vi "Straight Edge Detection subvi.vi"(8 "error in (no error)":errorcluster, 10 "ROI in":T2, 11 "Image in":T1(plugin-control)=refnum) -> (0 "error out":errorcluster, 1 "Solution Vector, y and x":dbl[](array[numeric]) format="%.2f", 2 "correct number of lines found = T":bool, 3 "Image":T1(plugin-control), 4 "edges found":i32)   [LabVIEW 2017]
doc: "This example shows how to use Find Straight Edges in NI Vision. Find Straight Edges finds lines (or straight edges) within a search region. Find Straight Edges is a precursor function to many of the gauging and inspection tasks. For example, the location of the straight edges found within a region that encloses an object can interpreted as the boundaries of the object whose dimensions have to be measured for a gauging application or the presence of a crack in the surface of an object for an inspection application."
uses:
  <vilib>/vision/NI_Vision_Development_Module.lvlib
panel:
  out "Straight Edges":T3(array[cluster])=[{"Point1 (Pixels)"={"X"=692.82367, "Y"=439.5}, "Point2 (Pixels)"={"X"=689.4538, "Y"=536.0}, "Point1 (Real-World)"={"X"=692.82367, "Y"=439.5}, "Point2 (Real-World)"={"X"=689.4538, "Y"=536.0}, "Angle (Pixel)"=-1.9999999999996223, "Angle (Real-World)"=-1.9999999999996223, "Score"=309.80392156862746, "Straightness"=0.0, "Average SNR (db)"=291.0237373163493, "Calibration Valid"=TRUE}, {"Point1 (Pixels)"={"X"=689.4637, "Y"=439.5}, "Point2 (Pixels)"={"X"=684.4063, "Y"=536.0}, "Point1 (Real-World)"={"X"=689.4637, "Y"=439.5}, "Point2 (Real-World)"={"X"=684.4063, "Y"=536.0}, "Angle (Pixel)"=-2.9999999999994333, "Angle (Real-World)"=-2.9999999999994333, "Score"=290.19607843137254, "Straightness"=0.0, "Average SNR (db)"=290.45582988516, "Calibration Valid"=TRUE}] {"Point2 (Real-World)"."Y" format="%.2f"; "Point2 (Real-World)"."X" format="%.2f"; "Point1 (Real-World)"."Y" format="%.2f"; "Point1 (Real-World)"."X" format="%.2f"; "Point2 (Pixels)"."Y" format="%.2f"; "Point2 (Pixels)"."X" format="%.2f"; "Point1 (Pixels)"."Y" format="%.2f"; "Point1 (Pixels)"."X" format="%.2f"}
  in  "Line Options":T4={"Number of Lines"=2, "Type"=4, "Minimum Score"=100.0, "Maximum Score"=1024.0, "Orientation"=0.0, "Angle Range"=10.0, "Angle Tolerance"=1.0, "Step Size"=3, "Min. SNR (db)"=0.0, "Min. Points (%)"=25.0, "Hough Iterations"=5} {"Min. Points (%)" min=0.0 max=100.0; "Min. SNR (db)" min=0.0; "Maximum Score" min=0.0 max=1024.0; "Minimum Score" min=1.0 max=1024.0 step=1.0; "Type" items=["First Edge Rake", "Best Edge Rake", "Hough Edge Rake", "First Edge Projection", "Best Edge Projection"]}
  in  "Edge Options":T5={"Edge Polarity"=0, "Kernel Size"=5, "Width"=3, "Minimum Edge Strength"=50.0, "Interpolation Type"=1, "Data Processing Method"=0} {"Data Processing Method" items=["Average", "Median"]; "Interpolation Type" items=["Zero Order"=0, "Bilinear"=1, "Bilinear Fixed"=4]; "Minimum Edge Strength" min=0.0 max=255.0 format="%.2g"; "Width" min=1 step=2; "Kernel Size" min=3 step=2; "Edge Polarity" items=["All Edges", "Rising Edges", "Falling Edges"]}
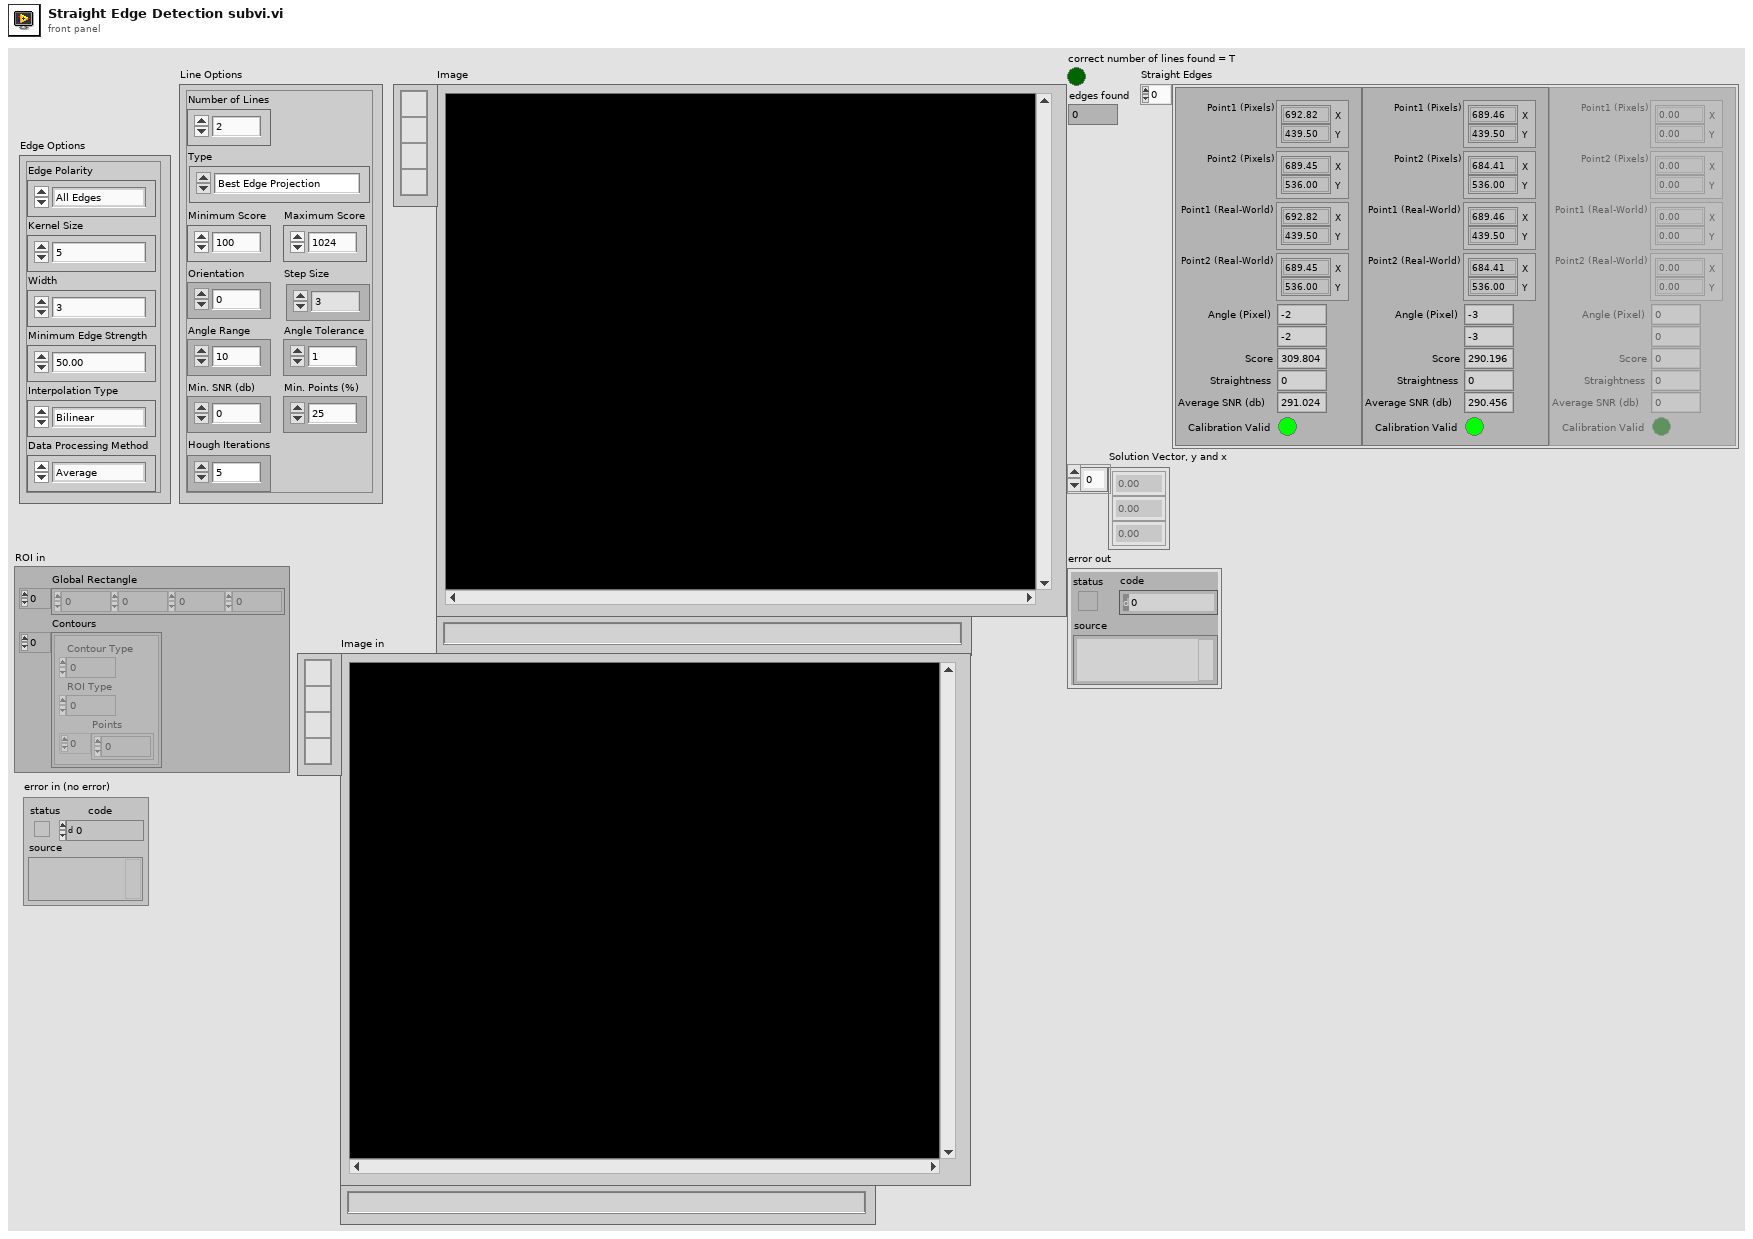
[diagram p1: front panel]
types:
  T1 = typedef "IMAQ Image.ctl" = refnum<image>
  T2 = cluster{"Global Rectangle":i32[], "Contours":cluster{"Contour Type":u32, "ROI Type":u32, "Points":i32[]}[]}
  T3 = cluster{"Point1 (Pixels)":cluster{"X":sgl, "Y":sgl}, "Point2 (Pixels)":cluster{"X":sgl, "Y":sgl}, "Point1 (Real-World)":cluster{"X":sgl, "Y":sgl}, "Point2 (Real-World)":cluster{"X":sgl, "Y":sgl}, "Angle (Pixel)":dbl, "Angle (Real-World)":dbl, "Score":dbl, "Straightness":dbl, "Average SNR (db)":dbl, "Calibration Valid":bool}[]
  T4 = cluster{"Number of Lines":i32, "Type":u16, "Minimum Score":dbl, "Maximum Score":dbl, "Orientation":dbl, "Angle Range":dbl, "Angle Tolerance":dbl, "Step Size":u32, "Min. SNR (db)":dbl, "Min. Points (%)":dbl, "Hough Iterations":i32}
  T5 = cluster{"Edge Polarity":u16, "Kernel Size":u32, "Width":u32, "Minimum Edge Strength":dbl, "Interpolation Type":u16, "Data Processing Method":u16}
  T6 = typedef "Search Line.ctl" = cluster{"Start Point":cluster{"X":sgl, "Y":sgl}, "End Point":cluster{"X":sgl, "Y":sgl}, "Edge Info":T7[], "Edge Map":dbl[], "Calibration Valid":bool}
  T7 = typedef "Edge New.ctl" = cluster{"Location (Pixel)":cluster{"X":sgl, "Y":sgl}, "Location (Real-World)":cluster{"X":sgl, "Y":sgl}, "Distance (Pixel)":dbl, "Distance (Real-World)":dbl, "Strength":dbl, "Noise":dbl, "Rising?":bool}
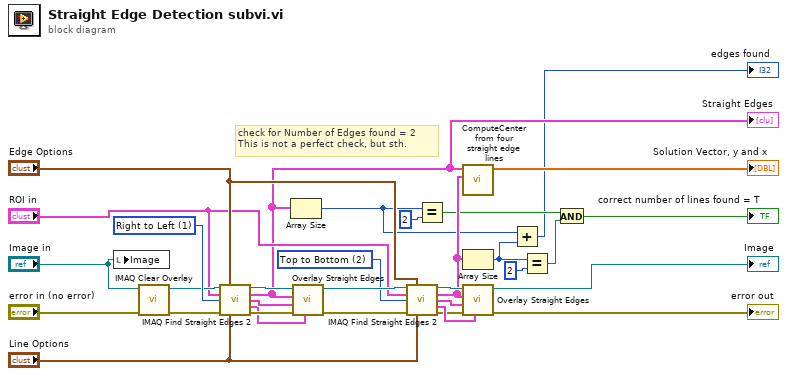
[diagram p0: block diagram]
diagram:
  w19 = u32 2 items=["Left to Right", "Right to Left", "Top to Bottom", "Bottom to Top"] ("Search Direction")
  w32 = u32 1 items=["Left to Right", "Right to Left", "Top to Bottom", "Bottom to Top"] ("Search Direction")
  # "check for Number of Edges found = 2\nThis is not a perfect check, but sth."
  n1 = local write "Image"("Image in") -> ()
  n2 = call "IMAQ Clear Overlay"("error in (no error)"="error in (no error)", "Image"="Image in") -> ("error out"=w31:errorcluster, "Image Out"=w30:T1)  [unwired: 8 in]
  n3 = call "IMAQ Find Straight Edges 2"("Image"=w30, "Edge Options"="Edge Options", "ROI Descriptor"="ROI in", "Search Direction"=w32, "error in (no error)"=w31, "Line Options"="Line Options") -> ("Image (duplicate)"=w29:T1, "Straight Edges"=w9:T3, "Search Lines Information"=w28:T6[], "Used Edges"=w26:cluster{"Edge Information":T7[]}[], "error out"=w27:errorcluster)  [unwired: 5 in]
  "Straight Edges" <- w9
  n4 = Array Size(array=w9) -> (size(s)=w2:i32)
  n5 = call "Overlay Straight Edges.vi"("All Edges (Pixel)"=w26, "error in"=w27, "Search Lines Information"=w28, "Straight Edges"=w9, "Image In"=w29) -> ("error out"=w20:errorcluster, "Image Out"=w21:T1)  [unwired: 5 in]
  n6 = call "IMAQ Find Straight Edges 2"("Image"=w21, "Edge Options"="Edge Options", "ROI Descriptor"="ROI in", "Search Direction"=w19, "error in (no error)"=w20, "Line Options"="Line Options") -> ("Image (duplicate)"=w22:T1, "Straight Edges"=w10:T3, "Search Lines Information"=w23:T6[], "Used Edges"=w25:cluster{"Edge Information":T7[]}[], "error out"=w24:errorcluster)  [unwired: 5 in]
  n7 = Equal?(x=w2, y=2) -> (x = y?=w5:bool)
  n8 = call "ComputeCenter from four straight edge lines.vi"("Straight Edges top to bottom"=w10, "Straight Edges Right to left"=w9) -> ("Solution Vector, y and x"=→"Solution Vector, y and x":dbl[])  [unwired: 9 in]
  n9 = Array Size(array=w10) -> (size(s)=w3:i32)
  n10 = call "Overlay Straight Edges.vi"("All Edges (Pixel)"=w25, "error in"=w24, "Search Lines Information"=w23, "Straight Edges"=w10, "Image In"=w22) -> ("error out"=→"error out":errorcluster, "Image Out"=→"Image":T1)  [unwired: 5 in]
  n11 = Add(x=w2, y=w3) -> (x+y=→"edges found":i32)
  n12 = Equal?(x=w3, y=2) -> (x = y?=w6:bool)
  n13 = And(x=w5, y=w6) -> (x .and. y?=→"correct number of lines found = T":bool)
